vi "FGV Ventile manuell schalten Crio.vi"(0 "Ventile schalten":u32, 9 "Ventilstellung":u32, 11 "error in (no error)":errorcluster caption="Fehler (Eingang, kein Fehler)", 13 "Aktion":T1) -> (4 "Ventile schalten":u32, 8 "Betrieb":u16, 10 "Ventilstellung":u32, 15 "error out":errorcluster caption="Fehler (Ausgang)")   [LabVIEW 2020, in "Anlagenuebersicht.lvlib"]
uses:
  Anlagenuebersicht.lvlib
  Aktion FGV Ventile manuell schalten Crio.ctl
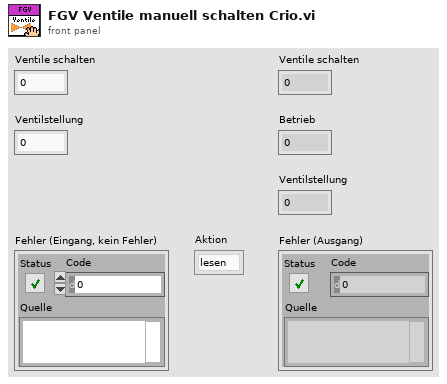
[diagram p1: front panel]
types:
  T1 = typedef "Anlagenuebersicht.lvlib/Aktion FGV Ventile manuell schalten Crio.ctl" = enum16{"lesen", "Ventile schalten", "Testbetrieb aktiv", "Testbetrieb inaktiv", "Anzeige Ventilstellung"}
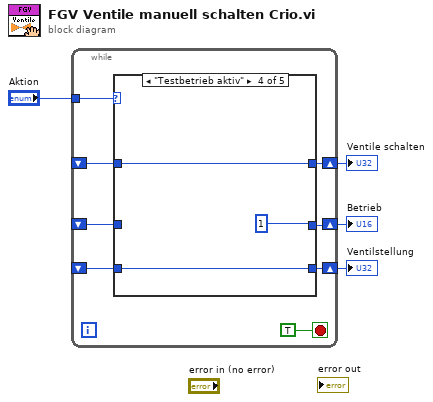
[diagram p0: block diagram]
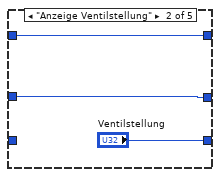
[diagram p3: hidden frame]
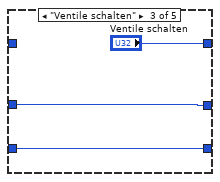
[diagram p4: hidden frame]
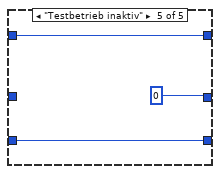
[diagram p5: hidden frame]
diagram:
  n1 = while {
    tunnel: "Aktion" -> [w11]
    shift-right: [w10] -> w3
    shift-left: _ -> [w9]
    shift-right: [w8] -> w2
    shift-left: _ -> [w7]
    shift-right: [w6] -> w1
    shift-left: _ -> [w5]
    stop <- TRUE stop-if-true
    n2 = case shown="\"Testbetrieb aktiv\"" w11 {
      tunnel: [w15 w18 "Ventile schalten" w24 w27] -> w10
      tunnel: w9 -> [w15 w18 _ w24 w27]
      tunnel: [w14 w17 w20 u16 1 ("Betrieb") u16 0 ("Betrieb")] -> w8
      tunnel: w7 -> [w14 w17 w20 _ _]
      tunnel: [w13 "Ventilstellung" w19 w22 w25] -> w6
      tunnel: w5 -> [w13 _ w19 w22 w25]
      frame "lesen", Default {
      }
      frame "Anzeige Ventilstellung" {
      }
      frame "Ventile schalten" {
      }
      frame "Testbetrieb aktiv" {
      }
      frame "Testbetrieb inaktiv" {
      }
    }
  }
  "Ventile schalten" <- w3
  "Betrieb" <- w2
  "Ventilstellung" <- w1
